vi "TDMSAdv addChannel.vi"(5 "channel name":string, 7 "group name (Untitled)":string, 8 "error in (no error)":errorcluster, 11 "TDMSAdv in":refnum<class "TDMSAdv.lvclass">) -> (0 "error out":errorcluster, 3 "TDMSAdv out":refnum<class "TDMSAdv.lvclass">)   [LabVIEW 2018, in "TDMSAdv.lvclass"]
uses:
  TDMSAdv.lvclass
  TDMSAdv.lvclass/TDMSAdv.ctl
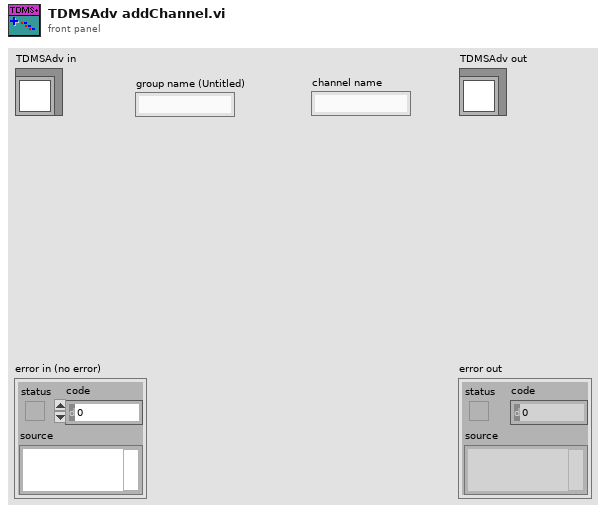
[diagram p1: front panel]
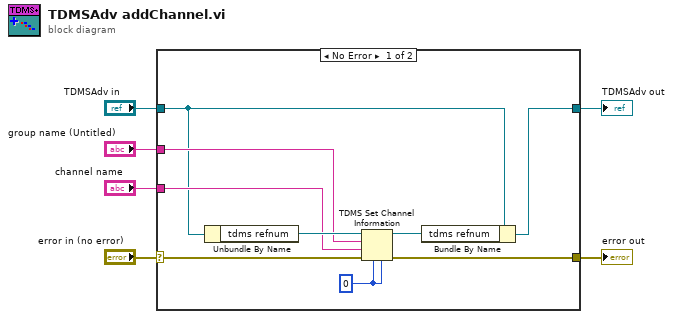
[diagram p0: block diagram]
diagram:
  n1 = case shown="No Error" "error in (no error)" {
    selector: "error in (no error)" -> [w12 w17]
    tunnel: [w11 w17] -> w5
    tunnel: [w7 w16] -> w3
    tunnel: "TDMSAdv in" -> [w9 w16]
    tunnel: "group name (Untitled)" -> [w14 _]
    tunnel: "channel name" -> [w13 _]
    frame No Error {
      w10 = u8 0 ("data type")
      n2 = Unbundle By Name(w9) -> ("tdms refnum"=w15:refnum<k34>)
      n3 = TDMS Set Channel Information(4:w10, 6:w10, 8:w12, 9:w13, 10:w14, 11:w15) -> (0:w11:errorcluster, 3:w8:refnum<k34>)  [unwired: 1 in]
      n4 = Bundle By Name(cluster=w9, "tdms refnum"=w8) -> (w7:refnum<class "TDMSAdv.lvclass">)
    }
    frame Error {
    }
  }
  "error out" <- w5
  "TDMSAdv out" <- w3
